vi "ShowHideProcessFrontPanel.vi"(7 "Hide / Show front panel":T1, 8 "error in (no error)":errorcluster, 11 "Process path":path) -> (0 "error out":errorcluster)   [LabVIEW 2011]
uses:
  Enum_HideShow_Process.ctl
  030 - EVENTS/06 - ToProcess/ToProcess_EnumCommand.ctl
  030 - EVENTS/06 - ToProcess/ToProcess.ctl
  030 - EVENTS/EnumFgvEventCommand.ctl
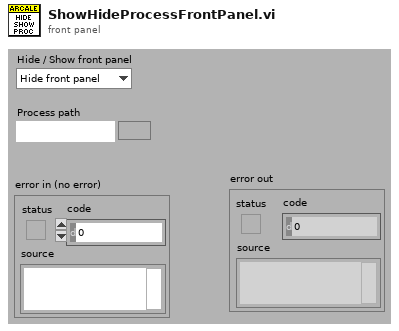
[diagram p1: front panel]
types:
  T1 = typedef "Enum_HideShow_Process.ctl" = enum16{"Hide front panel", "Show front panel"}
  T2 = typedef "ToProcess_EnumCommand.ctl" = enum16{"Show front panel", "Hide front panel"}
  T3 = typedef "ToProcess.ctl" = cluster{"Command":T2, "Process path":path}
  T4 = typedef "EnumFgvEventCommand.ctl" = enum16{"Setup", "Cleanup", "Get"}
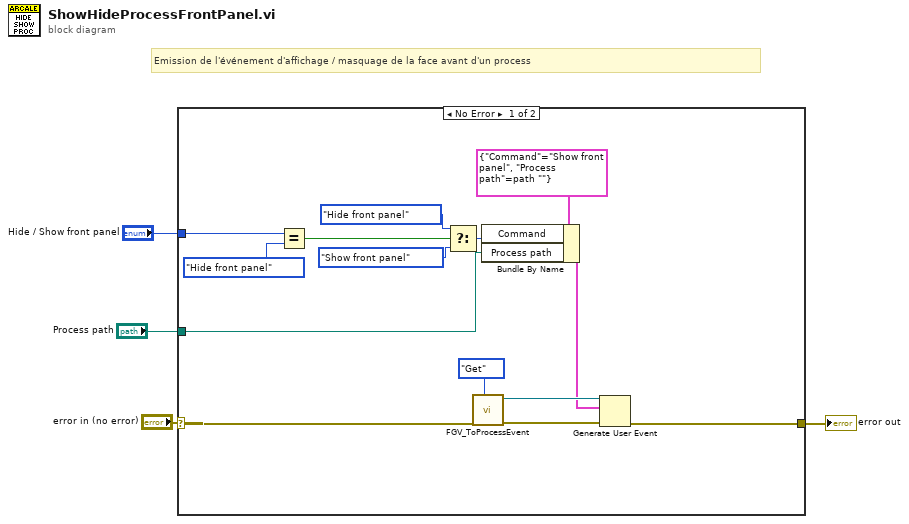
[diagram p0: block diagram]
diagram:
  # "Emission de l'événement d'affichage / masquage de la face avant d'un process"
  n1 = case shown="No Error" "error in (no error)" {
    selector: "error in (no error)" -> [w6 w19]
    tunnel: [w14 w19] -> w3
    tunnel: "Hide / Show front panel" -> [w8 _]
    tunnel: "Process path" -> [w5 _]
    frame No Error {
      n2 = Equal?(x=w8, y=Enum_HideShow_Process."Hide front panel") -> (x = y?=w11:bool)
      n3 = Select(t=ToProcess_EnumCommand."Hide front panel" ("Command"), s=w11, f=ToProcess_EnumCommand."Show front panel" ("Command")) -> (s? t:f=w7:T2)
      n4 = call "FGV_ToProcessEvent.vi"("Command"=EnumFgvEventCommand."Get", "error in (no error)"=w6) -> ("error out"=w17:errorcluster, "ToProcessEvent"=w16:refnum<user-event>)  [unwired: 8 in]
      n5 = Bundle By Name(cluster=T3 {"Command"=enum."Show front panel", "Process path"=path ""} ("event data"), "Command"=w7, "Process path"=w5) -> (w13:T3)
      n6 = Generate User Event(user event=w16, event data cluster=w13, error in=w17) -> (error out=w14:errorcluster)  [unwired: 1 out]
    }
    frame Error {
    }
  }
  "error out" <- w3
